vi "Get Measurement Metadata.vi"(8 "error in":errorcluster, 10 "service_class":string, 11 "project refnum":refnum<vi>) -> (0 "error out":errorcluster, 2 "default value":variant, 3 "metadata":T1)   [LabVIEW 2021, in "NI Measurement V2 Client Generator Runtime.lvlib"]
uses:
  NI Measurement V2 Client Generator Runtime.lvlib
  <vilib>/gRPC/Generated APIs/ni/measurementlink/measurement/v2/Measurement Service Client V2/RPC Messages/ni_measurementlink_measurement_v2_GetMetadataResponse.ctl
  <vilib>/gRPC/Generated APIs/ni/measurementlink/measurement/v2/Measurement Service Client V2/RPC Messages/ni_measurementlink_measurement_v2_MeasurementDetails.ctl
  <vilib>/gRPC/Generated APIs/ni/measurementlink/measurement/v2/Measurement Service Client V2/RPC Messages/ni_measurementlink_measurement_v2_MeasurementSignature.ctl
  <vilib>/gRPC/Generated APIs/ni/measurementlink/measurement/v2/Measurement Service Client V2/RPC Messages/ni_measurementlink_measurement_v2_ConfigurationParameter.ctl
  <vilib>/gRPC/Generated APIs/ni/measurementlink/measurement/v2/Measurement Service Client V2/RPC Messages/google_protobuf_Field_Kind.ctl
  <vilib>/gRPC/Generated APIs/ni/measurementlink/measurement/v2/Measurement Service Client V2/RPC Messages/ni_measurementlink_measurement_v2_ConfigurationParameter_AnnotationsEntry.ctl
  <vilib>/gRPC/Generated APIs/ni/measurementlink/measurement/v2/Measurement Service Client V2/RPC Messages/google_protobuf_Any.ctl
  <vilib>/gRPC/Generated APIs/ni/measurementlink/measurement/v2/Measurement Service Client V2/RPC Messages/ni_measurementlink_measurement_v2_Output.ctl
  <vilib>/gRPC/Generated APIs/ni/measurementlink/measurement/v2/Measurement Service Client V2/RPC Messages/ni_measurementlink_measurement_v2_Output_AnnotationsEntry.ctl
  <vilib>/gRPC/Generated APIs/ni/measurementlink/measurement/v2/Measurement Service Client V2/RPC Messages/ni_measurementlink_measurement_v2_UserInterfaceDetails.ctl
  <vilib>/gRPC/Generated APIs/ni/measurementlink/discovery/v1/RPC Messages/ni_measurementlink_discovery_v1_ResolveServiceRequest.ctl
  Client Generator Error Strings Global.vi
  <vilib>/gRPC/Generated APIs/ni/measurementlink/discovery/v1/ni.measurementlink.discovery.v1.api.lvlib
  <vilib>/gRPC/Generated APIs/ni/measurementlink/measurement/v2/Measurement Service Client V2/Measurement Service Client V2.lvlib
  <vilib>/Plug-In SDKs/Clients/Discovery V1/NI Discovery V1 Client.lvlib
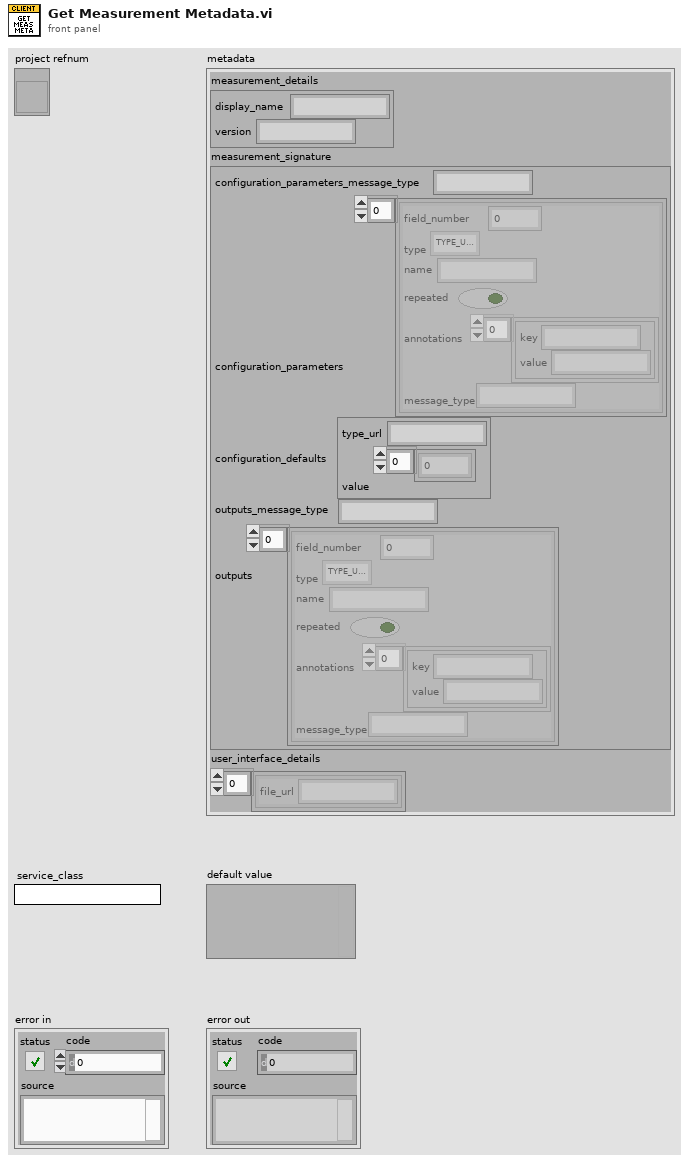
[diagram p1: front panel]
types:
  T1 = typedef "Measurement Service Client V2.lvlib/ni_measurementlink_measurement_v2_GetMetadataResponse.ctl" = cluster{"measurement_details":T2, "measurement_signature":T3, "user_interface_details":T10[]}
  T2 = typedef "Measurement Service Client V2.lvlib/ni_measurementlink_measurement_v2_MeasurementDetails.ctl" = cluster{"display_name":string, "version":string}
  T3 = typedef "Measurement Service Client V2.lvlib/ni_measurementlink_measurement_v2_MeasurementSignature.ctl" = cluster{"configuration_parameters_message_type":string, "configuration_parameters":T4[], "configuration_defaults":T7, "outputs_message_type":string, "outputs":T8[]}
  T4 = typedef "Measurement Service Client V2.lvlib/ni_measurementlink_measurement_v2_ConfigurationParameter.ctl" = cluster{"field_number":i32, "type":T5, "name":string, "repeated":bool, "annotations":T6[], "message_type":string}
  T5 = typedef "Measurement Service Client V2.lvlib/google_protobuf_Field_Kind.ctl" = enum32{"TYPE_UNKNOWN", "TYPE_DOUBLE", "TYPE_FLOAT", "TYPE_INT64", "TYPE_UINT64", "TYPE_INT32", "TYPE_FIXED64", "TYPE_FIXED32", "TYPE_BOOL", "TYPE_STRING", "TYPE_GROUP", "TYPE_MESSAGE", "TYPE_BYTES", "TYPE_UINT32", "TYPE_ENUM", "TYPE_SFIXED32", "TYPE_SFIXED64", "TYPE_SINT32", "TYPE_SINT64"}
  T6 = typedef "Measurement Service Client V2.lvlib/ni_measurementlink_measurement_v2_ConfigurationParameter_AnnotationsEntry.ctl" = cluster{"key":string, "value":string}
  T7 = typedef "Measurement Service Client V2.lvlib/google_protobuf_Any.ctl" = cluster{"type_url":string, "value":u8[]}
  T8 = typedef "Measurement Service Client V2.lvlib/ni_measurementlink_measurement_v2_Output.ctl" = cluster{"field_number":i32, "type":T5, "name":string, "repeated":bool, "annotations":T9[], "message_type":string}
  T9 = typedef "Measurement Service Client V2.lvlib/ni_measurementlink_measurement_v2_Output_AnnotationsEntry.ctl" = cluster{"key":string, "value":string}
  T10 = typedef "Measurement Service Client V2.lvlib/ni_measurementlink_measurement_v2_UserInterfaceDetails.ctl" = cluster{"file_url":string}
  T11 = typedef "ni.measurementlink.discovery.v1.api.lvlib/ni_measurementlink_discovery_v1_ResolveServiceRequest.ctl" = cluster{"provided_interface":string, "service_class":string, "deployment_target":string, "version":string}
  T12 = typedef "ni.measurementlink.discovery.v1.api.lvlib/ni_measurementlink_discovery_v1_ResolveServiceWithInformationResponse.ctl" = cluster{"service_location":T13, "service_descriptor":T14}
  T13 = typedef "ni.measurementlink.discovery.v1.api.lvlib/ni_measurementlink_discovery_v1_ServiceLocation.ctl" = cluster{"location":string, "insecure_port":string, "ssl_authenticated_port":string}
  T14 = typedef "ni.measurementlink.discovery.v1.api.lvlib/ni_measurementlink_discovery_v1_ServiceDescriptor.ctl" = cluster{"display_name":string, "description_url":string, "provided_interfaces":string[], "service_class":string, "annotations":T15[], "versions":string[]}
  T15 = typedef "ni.measurementlink.discovery.v1.api.lvlib/ni_measurementlink_discovery_v1_ServiceDescriptor_AnnotationsEntry.ctl" = cluster{"key":string, "value":string}
  T16 = typedef "grpc-lvsupport-release.lvlib/grpcId.ctl" = u64
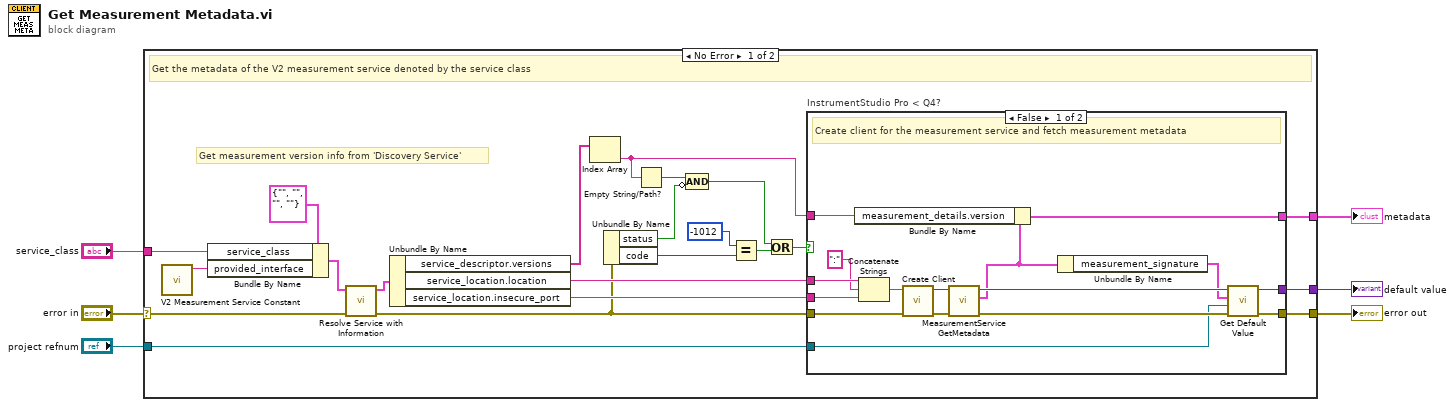
[diagram p0: block diagram]
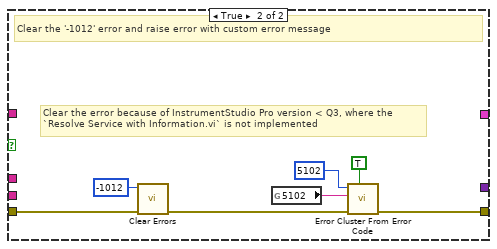
[diagram p2: hidden frame]
diagram:
  n1 = case shown="No Error" "error in" {
    selector: "error in" -> [w22 w52]
    tunnel: "service_class" -> [w28 _]
    tunnel: [w21 w52] -> w5
    tunnel: "project refnum" -> [w8 _]
    tunnel: [w20 _] -> w2
    tunnel: [w18 _] -> w1
    frame No Error {
      # "Get measurement version info from 'Discovery Service'"
      # "Get the metadata of the V2 measurement service denoted by the service class"
      n2 = call "V2 Measurement Service Constant.vi"() -> ("provided_interface"=w9:string)  [unwired: 11 in]
      n3 = Bundle By Name(cluster=T11 {"provided_interface"="", "service_class"="", "deployment_target"="", "version"=""} ("request data"), "service_class"=w28, "provided_interface"=w9) -> (w26:T11)
      n4 = call <vilib>:"Resolve Service with Information.vi"("error in"=w22, "request data"=w26) -> ("error out"=w17:errorcluster, "response data"=w25:T12)  [unwired: 8 in]
      n5 = Unbundle By Name(w25) -> ("service_descriptor.versions"=w19:string[], "service_location.location"=w24:string, "service_location.insecure_port"=w23:string)
      n6 = Index Array(array=w19) -> (element=w7:string)  [unwired: 1 in]
      n7 = Unbundle By Name(w17) -> ("status"=w14:bool, "code"=w15:i32)
      n8 = Empty String/Path?(string/path=w7) -> (empty?=w13:bool)
      n9 = Compound Arithmetic op=AND(w13, invert w14) -> (w10:bool)
      n10 = Equal?(x=-1012, y=w15) -> (x = y?=w11:bool)
      n11 = Or(x=w10, y=w11) -> (x .or. y?=w12:bool)
      n12 = case "InstrumentStudio Pro < Q4?" shown="False" w12 {
        tunnel: w17 -> [w41 w51]
        tunnel: w24 -> [w40 _]
        tunnel: w23 -> [w39 _]
        tunnel: [w36 w48] -> w21
        tunnel: [w33 _] -> w20
        tunnel: [w31 _] -> w18
        tunnel: w7 -> [w30 _]
        tunnel: w8 -> [w29 _]
        frame False {
          # "Create client for the measurement service and fetch measurement metadata"
          n13 = Concatenate Strings(w40, ":" ("string"), w39) -> (w42:string)
          n14 = call <vilib>:"Create Client.vi"("error in"=w41, "address"=w42) -> ("error out"=w43:errorcluster, "gRPC ID Out"=w44:T16)  [unwired: 8 in]
          n15 = call <vilib>:"MeasurementService GetMetadata.vi"("error in"=w43, "gRPC ID"=w44) -> ("error out"=w37:errorcluster, "Response Data"=w32:T1, "gRPC ID out"=w35:T16)  [unwired: 7 in]
          n16 = Bundle By Name(cluster=w32, "measurement_details.version"=w30) -> (w31:T1)
          n17 = Unbundle By Name(w32) -> ("measurement_signature"=w34:T3)
          n18 = call "Get Default Value.vi"("error in"=w37, "project refnum"=w29, "measurement_signature"=w34, "gRPCid in"=w35) -> ("error out"=w36:errorcluster, "default value"=w33:variant)  [unwired: 6 in]
        }
        frame True {
          # "Clear the error because of InstrumentStudio Pro version < Q3, where the \n`Resolve Service with Information.vi` is not implemented"
          # "Clear the '-1012' error and raise error with custom error message"
          n19 = call <vilib>:"Clear Errors.vi"("error in (no error)"=w51, "specific error code to clear (0: all)"=-1012) -> ("error out"=w50:errorcluster)  [unwired: 4 in, 1 out]
          n20 = global read "Client Generator Error Strings Global.vi" "5102"() -> (w45:string)
          n21 = call <vilib>:"Error Cluster From Error Code.vi"("show call chain? (False)"=TRUE, "error in (no error)"=w50, "error message (\"\")"=w45, "error code (0)"=5102) -> ("error out"=w48:errorcluster)  [unwired: 5 in]
        }
      }
    }
    frame Error {
      # "Pass"
    }
  }
  "error out" <- w5
  "metadata" <- w1
  "default value" <- w2
